vi "Player Info.vi"(11 "Explorer in":refnum<class "Explorer.lvclass">) -> (1 "Victory Speech":string, 2 "Name":string, 3 "Explorer out":refnum<class "Explorer.lvclass">)   [LabVIEW 2015, in "Explorer.lvclass"]
uses:
  Explorer.lvclass
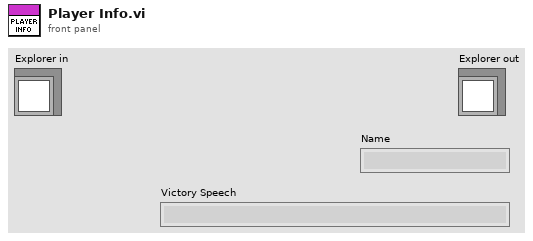
[diagram p1: front panel]
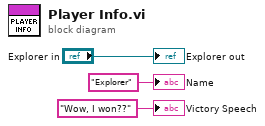
[diagram p0: block diagram]
diagram:
  "Explorer out" <- "Explorer in"
  "Name" <- "Explorer" ("Name")
  "Victory Speech" <- "Wow, I won??" ("Victory Speech")
